vi "Drive Train.vi"() -> ()   [LabVIEW 2018]
uses:
  <vilib>/Rock Robotics/SystemInterfaces/DIO/FPGA_DIOChannel.ctl
  <vilib>/Rock Robotics/SystemInterfaces/AI/FPGA_AIChannel.ctl
  <vilib>/Rock Robotics/WPI/ThirdParty/Sensors/navX/_TypeDefs/FRIC_navX_DeviceNumbersTypeDef.ctl
  <vilib>/Rock Robotics/WPI/DriverStation/WPI_DriverStationRobotMode2.ctl
  <vilib>/Rock Robotics/WPI/ThirdParty/Phoenix-LabVIEW/Motor Controller/Controls/CTRE_Phoenix_MotorControl_NeutralMode.ctl
  <vilib>/Rock Robotics/WPI/Counter/WPI_CounterDigitalInputToDigitalSource.vi
  Times/Times Global.vi
  Drive Train Global.vi
  Robot Global Data.vi
  <vilib>/ptbypt/NI_PtbyPt.lvlib
panel:
  out "Cont Yaw Zero":dbl
  out "Loop 2":u32=30
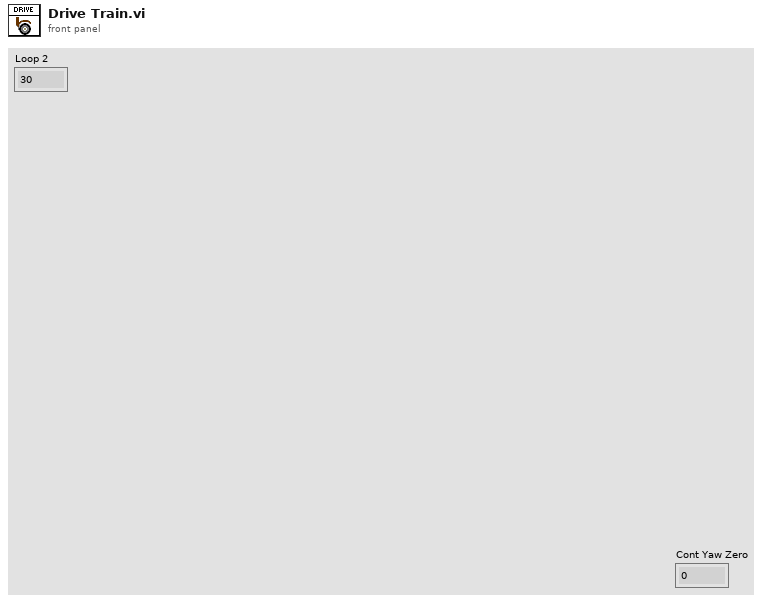
[diagram p1: front panel]
types:
  T1 = typedef "FPGA_AIChannel.ctl" = enum8{"AI 0", "AI 1", "AI 2", "AI 3", "AI MXP 0", "AI MXP 1", "AI MXP 2", "AI MXP 3", "Invalid"}
  T2 = typedef "FPGA_DIOChannel.ctl" = enum8{"DIO 0", "DIO 1", "DIO 2", "DIO 3", "DIO 4", "DIO 5", "DIO 6", "DIO 7", "DIO 8", "DIO 9", "DIO MXP 0", "DIO MXP 1", "DIO MXP 2", "DIO MXP 3", "DIO MXP 4", "DIO MXP 5", "DIO MXP 6", "DIO MXP 7", "DIO MXP 8", "DIO MXP 9", "DIO MXP 10", "DIO MXP 11", "DIO MXP 12", "DIO MXP 13", "DIO MXP 14", "DIO MXP 15", "SPI Port CS1", "SPI Port CS2", "SPI Port CS3", "SPI Port MISO", "SPI Port MOSI", "Invalid"}
  T3 = typedef "FRIC_navX_DeviceNumbersTypeDef.ctl" = enum16{"Dev0", "Dev1", "Dev2", "Dev3"}
  T4 = cluster{"Rollover":dbl, "Yaw":dbl, "Cont Yaw":dbl}
  T5 = typedef "CTRE_Phoenix_MotorControl_NeutralMode.ctl" = enum8{"EEPROMSetting", "Override to Coast", "Override to Brake"}
  T6 = typedef "WPI_MotorControlDeviceRef.ctl" = cluster{"DeviceStatus":errorcluster, "Type":T7, "PWM":cluster{"PWM Channel":T8, "DeadBand":T9}, "CAN":cluster{"Device Number":u8, "SetOutput VI Ref":variant, "GetOutput VI Ref":variant, "Enable VI Ref":variant, "Disable VI Ref":variant, "Data":variant}, "Invert":bool, "DIO PWM":cluster{"PWM \"Enable\" Channel":T8, "DIOChannel":T2, "PWM Rate":dbl}}
  T7 = typedef "WPI_MotorControlType.ctl" = enum16{"PWM", "CAN", "DIO PWM"}
  T8 = typedef "FPGA_DIOPWMChannel.ctl" = enum8{"PWM 0", "PWM 1", "PWM 2", "PWM 3", "PWM 4", "PWM 5", "PWM 6", "PWM 7", "PWM 8", "PWM 9", "PWM MXP 0", "PWM MXP 1", "PWM MXP 2", "PWM MXP 3", "PWM MXP 4", "PWM MXP 5", "PWM MXP 6", "PWM MXP 7", "PWM MXP 8", "PWM MXP 9", "Invalid"}
  T9 = typedef "WPI_PWMDeadband.ctl" = cluster{"Name":string, "maxPositivePwm":i32, "minPositivePwm":i32, "centerPwm":i32, "maxNegativePwm":i32, "minNegativePwm":i32, "angularRange":u16}
  T10 = typedef "WPI_DigitalInputDevRef.ctl" = cluster{"DevStatus":errorcluster, "DIO Channel":T2}
  T11 = typedef "WPI_PotentiometerDevRef.ctl" = cluster{"DevStatus":errorcluster, "Analog Channel":T1, "Invert Output":bool}
  T12 = typedef "FPGA_CounterEncoderSourceConvertionLVSourceType.ctl" = cluster{"DevStatus":errorcluster, "AnalogTriggerMode?":bool, "DigitalMode":cluster{"DIO Channel":T13}, "AnalogTriggerMode":cluster{"AnalogTriggerIndex":T14, "OutputType":T15}}
  T13 = typedef "FPGA_DIODigitalSourceChannel.ctl" = enum8{"DIO 0", "DIO 1", "DIO 2", "DIO 3", "DIO 4", "DIO 5", "DIO 6", "DIO 7", "DIO 8", "DIO 9", "DIO MXP 0", "DIO MXP 1", "DIO MXP 2", "DIO MXP 3", "DIO MXP 4", "DIO MXP 5", "DIO MXP 6", "DIO MXP 7", "DIO MXP 8", "DIO MXP 9", "DIO MXP 10", "DIO MXP 11", "DIO MXP 12", "DIO MXP 13", "DIO MXP 14", "DIO MXP 15", "SPI Port CS1", "SPI Port CS2", "SPI Port CS3", "SPI Port MISO", "SPI Port MOSI", "Disabled"}
  T14 = typedef "FPGA_AnalogTriggerIndex.ctl" = enum8{"Trig 0", "Trig 1", "Trig 2", "Trig 3", "Trig 4", "Trig 5", "Trig 6", "Trig 7", "Invalid"}
  T15 = typedef "FPGA_AnalogTriggerOutType.ctl" = enum16{"InWindow", "TriggerState", "Rising", "Falling"}
  T16 = typedef "WPI_EncoderDevRef.ctl" = cluster{"DevStatus":errorcluster, "EncoderIndex":T17, "CounterIndex":T18, "DistancePerCount":dbl, "Decoding Type":T19}
  T17 = typedef "FPGA_EncoderIdx.ctl" = enum8{"Enc 0", "Enc 1", "Enc 2", "Enc 3", "Enc 4", "Enc 5", "Enc 6", "Enc 7", "Invalid"}
  T18 = typedef "FPGA_CounterCtrSystemIndex.ctl" = enum8{"Ctr 0", "Ctr 1", "Ctr 2", "Ctr 3", "Ctr 4", "Ctr 5", "Ctr 6", "Ctr 7", "Invalid"}
  T19 = typedef "WPI_EncoderType.ctl" = enum16{"1x", "2x", "4x"}
  T20 = typedef "WPI_DriverStationRobotMode2.ctl" = enum16{"Autonomous Disabled", "Autonomous Enabled", "Teleop Disabled", "Teleop Enabled", "Disconnected", "Finish", "Test Disabled", "Test Enabled", "Emergency Stopped"}
  T21 = cluster{"FrontLeft":dbl, "FrontRight":dbl, "BackLeft":dbl, "BackRight":dbl}
  T22 = enum16{"Back Left", "Back Right", "Front Left", "Front Right"}
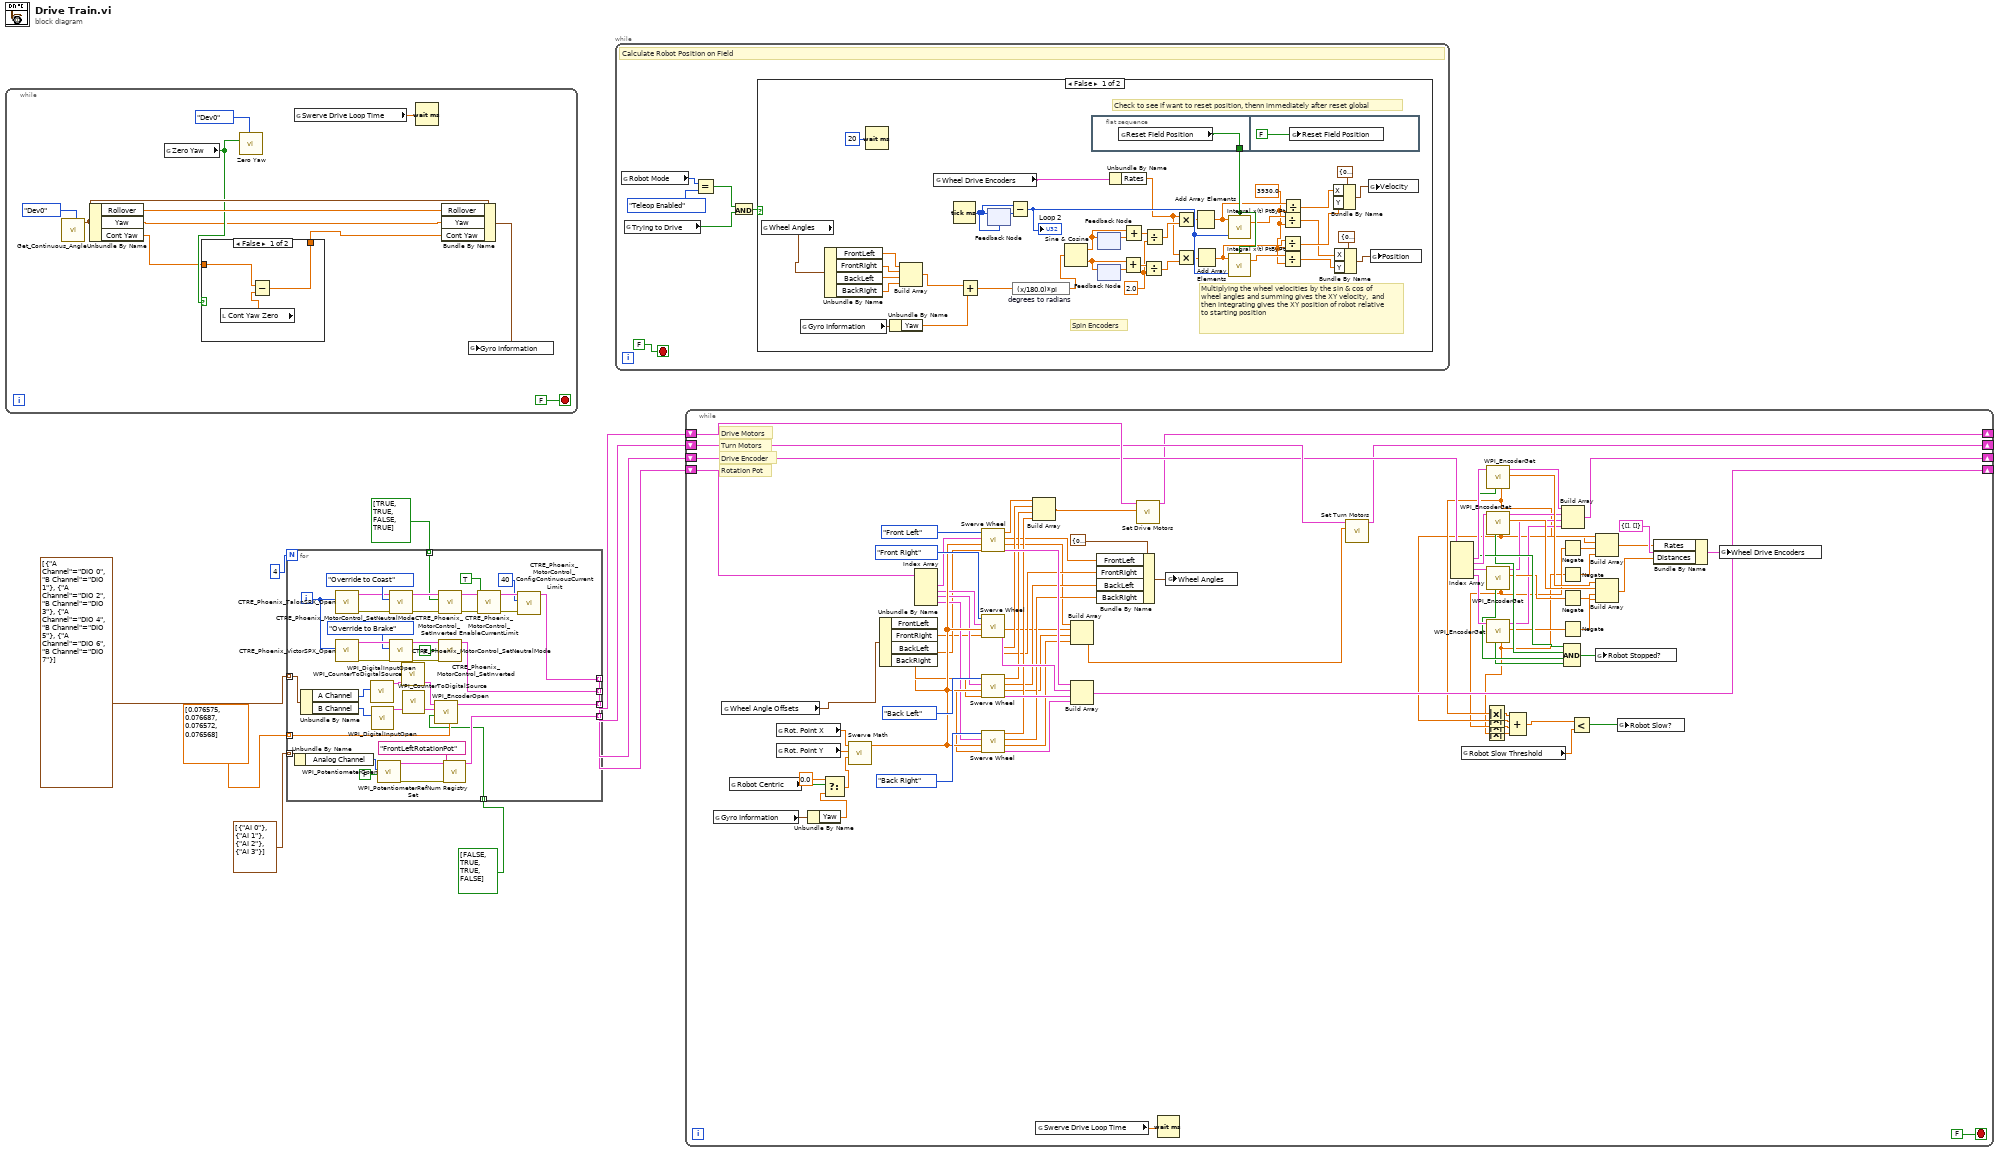
[diagram p0: block diagram]
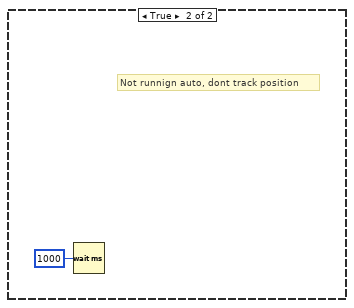
[diagram p2: hidden frame]
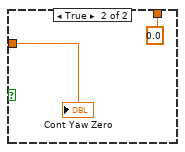
[diagram p3: hidden frame]
diagram:
  n1 = while {
    stop <- FALSE stop-if-true
    n2 = call <vilib>:"Get_Continuous_Angle.vi"("Device Number"=FRIC_navX_DeviceNumbersTypeDef."Dev0") -> ("Continuous Angle"=w15:T4)  [unwired: 10 in]
    n3 = Unbundle By Name(w15) -> ("Rollover"=w16:dbl, "Yaw"=w12:dbl, "Cont Yaw"=w13:dbl)
    n4 = global read "Drive Train Global.vi" "Zero Yaw"() -> (w14:bool)
    n5 = case shown="False" w14 {
      tunnel: w13 -> [w24 w26]
      tunnel: [w23 0.0] -> w11
      frame False {
        n6 = local read "Cont Yaw Zero"() -> (w22:dbl)
        n7 = Subtract(x=w24, y=w22) -> (x-y=w23:dbl)
      }
      frame True {
        "Cont Yaw Zero" <- w26
      }
    }
    n8 = call <vilib>:"Zero Yaw.vi"("Device Number"=FRIC_navX_DeviceNumbersTypeDef."Dev0", "Zero"=w14) -> ()  [unwired: 10 in]
    n9 = global read "Times Global.vi" "Swerve Drive Loop Time"() -> (w19:dbl)
    n10 = Wait (ms)(milliseconds to wait=w19) -> ()  [unwired: 1 out]
    n11 = Bundle By Name(cluster=w15, "Rollover"=w16, "Yaw"=w12, "Cont Yaw"=w11) -> (w17:T4)
    n12 = global write "Drive Train Global.vi" "Gyro Information"(w17) -> ()
  }
  n13 = for {
    N: 4 -> [_]
    tunnel: cluster{"A Channel":T2, "B Channel":T2}[] [{"A Channel"=enum."DIO 0", "B Channel"=enum."DIO 1"}, {"A Channel"=enum."DIO 2", "B Channel"=enum."DIO 3"}, {"A Channel"=enum."DIO 4", "B Channel"=enum."DIO 5"}, {"A Channel"=enum."DIO 6", "B Channel"=enum."DIO 7"}] -> [w44] mode=indexing
    tunnel: cluster{"Analog Channel":T1}[] [{"Analog Channel"=enum."AI 0"}, {"Analog Channel"=enum."AI 1"}, {"Analog Channel"=enum."AI 2"}, {"Analog Channel"=enum."AI 3"}] -> [w41] mode=indexing
    tunnel: dbl[] [0.076575, 0.076687, 0.076572, 0.076568] -> [w39] mode=indexing
    tunnel: [w28] -> w6 mode=indexing
    tunnel: [w38] -> w5 mode=indexing
    tunnel: [w37] -> w4 mode=indexing
    tunnel: [w36] -> w3 mode=indexing
    tunnel: bool[] [TRUE, TRUE, FALSE, TRUE] -> [w35] mode=indexing
    tunnel: bool[] [FALSE, TRUE, TRUE, FALSE] -> [w27] mode=indexing
    i -> [w45]
    n14 = Unbundle By Name(w41) -> ("Analog Channel"=w40:T1)
    n15 = Unbundle By Name(w44) -> ("A Channel"=w43:T2, "B Channel"=w42:T2)
    n16 = call <vilib>:"CTRE_Phoenix_TalonSRX_Open.vi"("Device Number"=w45) -> ("error out"=w46:errorcluster, "CAN Talon SRX Ref"=w47:T6)  [unwired: 9 in]
    n17 = call <vilib>:"CTRE_Phoenix_VictorSPX_Open.vi"("Device Number"=w45) -> ("error out"=w56:errorcluster, "CAN Talon SRX Ref"=w55:T6)  [unwired: 9 in]
    n18 = call <vilib>:"WPI_DigitalInputOpen.vi"("DIO Channel"=w43) -> ("DigitalInputDevRef"=w63:T10)  [unwired: 1 in, 9 out]
    n19 = call <vilib>:"WPI_DigitalInputOpen.vi"("DIO Channel"=w42) -> ("DigitalInputDevRef"=w62:T10)  [unwired: 1 in, 9 out]
    n20 = call <vilib>:"WPI_PotentiometerOpen.vi"("Invert Output"=FALSE, "Analog Channel"=w40) -> ("error out"=w58:errorcluster, "PotDevRef"=w59:T11)  [unwired: 8 in]
    n21 = call <vilib>:"CTRE_Phoenix_MotorControl_SetNeutralMode.vi"("error in (no error)"=w46, "Motor Control Neutral Mode"=CTRE_Phoenix_MotorControl_NeutralMode."Override to Coast", "PhoenixMotorControlDevRef"=w47) -> ("error out"=w49:errorcluster, "PhoenixMotorControlDevRef"=w50:T6)  [unwired: 7 in]
    n22 = call <vilib>:"CTRE_Phoenix_MotorControl_SetNeutralMode.vi"("error in (no error)"=w56, "Motor Control Neutral Mode"=CTRE_Phoenix_MotorControl_NeutralMode."Override to Brake", "PhoenixMotorControlDevRef"=w55) -> ("error out"=w53:errorcluster, "PhoenixMotorControlDevRef"=w52:T6)  [unwired: 7 in]
    n23 = call-poly <vilib>:"WPI_CounterToDigitalSource.vi"("DigitalInputDevRef"=w63) -> ("Digital Source"=w64:T12)  [unwired: 6 out]
    n24 = call-poly <vilib>:"WPI_CounterToDigitalSource.vi"("DigitalInputDevRef"=w62) -> ("Digital Source"=w61:T12)  [unwired: 6 out]
    n25 = call <vilib>:"WPI_EncoderOpen.vi"("DistancePerCount"=w39, "Invert Direction (False)"=w27, "BSource"=w61, "ASource"=w64) -> ("EncoderDevRef"=w37:T16)  [unwired: 4 in, 3 out]
    n26 = call <vilib>:"CTRE_Phoenix_MotorControl_SetInverted.vi"("error in (no error)"=w49, "Invert?"=w35, "PhoenixMotorControlDevRef"=w50) -> ("error out"=w34:errorcluster, "PhoenixMotorControlDevRef"=w33:T6)  [unwired: 7 in]
    n27 = call <vilib>:"CTRE_Phoenix_MotorControl_SetInverted.vi"("error in (no error)"=w53, "Invert?"=FALSE, "PhoenixMotorControlDevRef"=w52) -> ("PhoenixMotorControlDevRef"=w38:T6)  [unwired: 7 in, 1 out]
    n28 = call <vilib>:"WPI_PotentiometerRefNum Registry Set.vi"("error in (no error)"=w58, "refnum name"="FrontLeftRotationPot", "PotDevRef"=w59) -> ("PotDevRef"=w36:T11)  [unwired: 7 in, 1 out]
    n29 = call <vilib>:"CTRE_Phoenix_MotorControl_EnableCurrentLimit.vi"("error in (no error)"=w34, "Enable Current Limit?"=TRUE, "PhoenixMotorControlDevRef"=w33) -> ("error out"=w31:errorcluster, "PhoenixMotorControlDevRef"=w30:T6)  [unwired: 7 in]
    n30 = call <vilib>:"CTRE_Phoenix_MotorControl_ConfigContinuousCurrentLimit.vi"("error in (no error)"=w31, "Continuous Current Limit (Amps)"=40, "PhoenixMotorControlDevRef"=w30) -> ("PhoenixMotorControlDevRef"=w28:T6)  [unwired: 7 in, 1 out]
  }
  n31 = while {
    stop <- FALSE stop-if-true
    # "Calculate Robot Position on Field"
    n32 = global read "Robot Global Data.vi" "Robot Mode"() -> (w69:T20)
    n33 = global read "Robot Global Data.vi" "Trying to Drive"() -> (w66:bool)
    n34 = Equal?(x=w69, y=WPI_DriverStationRobotMode2."Teleop Enabled") -> (x = y?=w65:bool)
    n35 = And(x=w65, y=w66) -> (x .and. y?=w67:bool)
    n36 = case shown="False" w67 {
      frame False {
        w90 = 3930.0 ("y")
        w100 = 2.0
        # "Check to see if want to reset position, thenn immediately after reset global"
        # "Spin Encoders"
        # "Multiplying the wheel velocities by the sin & cos of wheel angles and summing gives the XY velocity,  and then integrating gives the XY position of robot relative to starting position"
        n37 = global read "Drive Train Global.vi" "Wheel Angles"() -> (w88:T21)
        n38 = global read "Drive Train Global.vi" "Gyro Information"() -> (w81:T4)
        n39 = Unbundle By Name(w88) -> ("FrontLeft"=w87:dbl, "FrontRight"=w86:dbl, "BackLeft"=w85:dbl, "BackRight"=w84:dbl)
        n40 = Wait (ms)(milliseconds to wait=u32 20) -> ()  [unwired: 1 out]
        n41 = Unbundle By Name(w81) -> ("Yaw"=w80:dbl)
        n42 = Build Array(w87, w86, w85, w84) -> (w83:dbl[])
        n43 = global read "Drive Train Global.vi" "Wheel Drive Encoders"() -> (w82:cluster{"Rates":dbl[], "Distances":dbl[]})
        n44 = Tick Count (ms)() -> (millisecond timer value=w96:u32)
        n45 = Add(x=w83, y=w80) -> (x+y=w89:dbl[])
        n46 = feedback #1(w96) -> (w111:u32)
        n47 = feedback-in #1(w96) -> ()
        n48 = Subtract(x=w96, y=w111) -> (x-y=w110:u32)
        "Loop 2" <- w110
        n49 = expression code="(x/180.0)*pi" "degrees to radians"(w89) -> (w95:dbl[])
        n50 = Sine & Cosine(0:w95) -> (1:w106:dbl[], 2:w101:dbl[])
        n51 = flat-sequence {
          tunnel: [w112] -> w98
          frame #0 {
            n52 = global read "Drive Train Global.vi" "Reset Field Position"() -> (w112:bool)
          }
          frame #1 {
            n53 = global write "Drive Train Global.vi" "Reset Field Position"(FALSE) -> ()
          }
        }
        n54 = feedback #2() -> (w107:dbl[])  [unwired: 1 in]
        n55 = feedback-in #2(w106) -> ()
        n56 = feedback #3() -> (w102:dbl[])  [unwired: 1 in]
        n57 = feedback-in #3(w101) -> ()
        n58 = Unbundle By Name(w82) -> ("Rates"=w97:dbl[])
        n59 = Add(x=w101, y=w102) -> (x+y=w103:dbl[])
        n60 = Add(x=w106, y=w107) -> (x+y=w104:dbl[])
        n61 = Divide(x=w103, y=w100) -> (x/y=w99:dbl[])
        n62 = Divide(x=w104, y=w100) -> (x/y=w105:dbl[])
        n63 = Multiply(x=w97, y=w105) -> (x*y=w109:dbl[])
        n64 = Multiply(x=w97, y=w99) -> (x*y=w108:dbl[])
        n65 = Add Array Elements(numeric array=w109) -> (sum=w93:dbl)
        n66 = Add Array Elements(numeric array=w108) -> (sum=w92:dbl)
        n67 = call <vilib>:"Integral x(t) PtByPt.vi"("initialize"=w98, "dt"=w110, "x"=w93) -> ("integral x(t)"=w94:dbl)  [unwired: 1 in, 1 out]
        n68 = call <vilib>:"Integral x(t) PtByPt.vi"("initialize"=w98, "dt"=w110, "x"=w92) -> ("integral x(t)"=w91:dbl)  [unwired: 1 in, 1 out]
        n69 = Divide(x=w94, y=w90) -> (x/y=w74:dbl)
        n70 = Divide(x=w92, y=w90) -> (x/y=w77:dbl)
        n71 = Divide(x=w91, y=w90) -> (x/y=w73:dbl)
        n72 = Divide(x=w93, y=w90) -> (x/y=w79:dbl)
        n73 = Bundle By Name(cluster=cluster{"X":dbl, "Y":dbl} {"X"=0.0, "Y"=0.0} ("Position"), "X"=w79, "Y"=w77) -> (w71:cluster{"X":dbl, "Y":dbl})
        n74 = Bundle By Name(cluster=cluster{"X":dbl, "Y":dbl} {"X"=0.0, "Y"=0.0} ("Position"), "X"=w74, "Y"=w73) -> (w75:cluster{"X":dbl, "Y":dbl})
        n75 = global write "Drive Train Global.vi" "Velocity"(w71) -> ()
        n76 = global write "Drive Train Global.vi" "Position"(w75) -> ()
      }
      frame True {
        # "Not runnign auto, dont track position"
        n77 = Wait (ms)(milliseconds to wait=u32 1000) -> ()  [unwired: 1 out]
      }
    }
  }
  n78 = while {
    shift-right: [w195] -> _
    shift-left: w6 -> [w199]
    shift-right: [w194] -> _
    shift-left: w5 -> [w198]
    shift-right: [w193] -> _
    shift-left: w4 -> [w197]
    shift-right: [w192] -> _
    shift-left: w3 -> [w196]
    stop <- FALSE stop-if-true
    # "Rotation Pot"
    # "Drive Encoder"
    # "Turn Motors"
    # "Drive Motors"
    n79 = global read "Drive Train Global.vi" "Gyro Information"() -> (w186:T4)
    n80 = global read "Drive Train Global.vi" "Wheel Angle Offsets"() -> (w153:T21)
    n81 = global read "Drive Train Global.vi" "Robot Centric"() -> (w156:bool)
    n82 = global read "Drive Train Global.vi" "Rot. Point X"() -> (w185:dbl)
    n83 = global read "Drive Train Global.vi" "Rot. Point Y"() -> (w184:dbl)
    n84 = Unbundle By Name(w186) -> ("Yaw"=w154:dbl)
    n85 = Select(t=0.0, s=w156, f=w154) -> (s? t:f=w157:dbl)
    n86 = call "Swerve Math.vi"("Yaw"=w157, "Rot. Point Y"=w184, "Rot. Point X"=w185) -> ("Swerve Math Ouput"=w187:dbl[])  [unwired: 8 in]
    n87 = Unbundle By Name(w153) -> ("FrontLeft"=w161:dbl, "FrontRight"=w160:dbl, "BackLeft"=w159:dbl, "BackRight"=w158:dbl)
    n88 = Index Array(array=w196) -> (element #1=w183:T11, element #2=w182:T11, element #3=w181:T11, element #4=w180:T11)  [unwired: 4 in]
    n89 = call "Swerve Wheel.vi"("Wheel Angle Offset"=w161, "Inputs"=w187, "Pot Ref In"=w183, "Wheel"=T22."Front Left") -> ("Pot Ref Out"=w176:T11, "Motor Output"=w165:dbl, "Wheel Angle"=w170:dbl, "Speed"=w175:dbl)  [unwired: 4 in]
    n90 = call "Swerve Wheel.vi"("Wheel Angle Offset"=w160, "Inputs"=w187, "Pot Ref In"=w182, "Wheel"=T22."Front Right") -> ("Pot Ref Out"=w177:T11, "Motor Output"=w164:dbl, "Wheel Angle"=w169:dbl, "Speed"=w174:dbl)  [unwired: 4 in]
    n91 = call "Swerve Wheel.vi"("Wheel Angle Offset"=w159, "Inputs"=w187, "Pot Ref In"=w181, "Wheel"=T22."Back Left") -> ("Pot Ref Out"=w178:T11, "Motor Output"=w163:dbl, "Wheel Angle"=w168:dbl, "Speed"=w173:dbl)  [unwired: 4 in]
    n92 = call "Swerve Wheel.vi"("Wheel Angle Offset"=w158, "Inputs"=w187, "Pot Ref In"=w180, "Wheel"=T22."Back Right") -> ("Pot Ref Out"=w179:T11, "Motor Output"=w162:dbl, "Wheel Angle"=w167:dbl, "Speed"=w172:dbl)  [unwired: 4 in]
    n93 = Build Array(w175, w174, w173, w172) -> (w151:dbl[])
    n94 = global read "Times Global.vi" "Swerve Drive Loop Time"() -> (w200:dbl)
    n95 = Build Array(w165, w164, w163, w162) -> (w152:dbl[])
    n96 = Build Array(w176, w177, w178, w179) -> (w192:T11[])
    n97 = Bundle By Name(cluster=T21 {"FrontLeft"=0.0, "FrontRight"=0.0, "BackLeft"=0.0, "BackRight"=0.0} ("Wheel Angles"), "FrontLeft"=w170, "FrontRight"=w169, "BackLeft"=w168, "BackRight"=w167) -> (w166:T21)
    n98 = call "Set Drive Motors.vi"("appended array"=w151, "Motors In"=w199) -> ("Motors Out"=w195:T6[])  [unwired: 9 in]
    n99 = Wait (ms)(milliseconds to wait=w200) -> ()  [unwired: 1 out]
    n100 = global write "Drive Train Global.vi" "Wheel Angles"(w166) -> ()
    n101 = call "Set Turn Motors.vi"("appended array"=w152, "Motors In"=w198) -> ("Motors Out"=w194:T6[])  [unwired: 9 in]
    n102 = Index Array(array=w197) -> (element #1=w150:T16, element #2=w149:T16, element #3=w148:T16, element #4=w147:T16)  [unwired: 4 in]
    n103 = global read "Drive Train Global.vi" "Robot Slow Threshold"() -> (w115:dbl)
    n104 = call <vilib>:"WPI_EncoderGet.vi"("EncoderDevRef"=w150) -> ("Distance"=w130:dbl, "EncoderDevRef"=w129:T16, "Rate"=w120:dbl, "Stopped"=w141:bool)  [unwired: 5 in, 2 out]
    n105 = Absolute Value(x=w120) -> (abs(x)=w124:dbl)
    n106 = call <vilib>:"WPI_EncoderGet.vi"("EncoderDevRef"=w149) -> ("Distance"=w134:dbl, "EncoderDevRef"=w128:T16, "Rate"=w119:dbl, "Stopped"=w140:bool)  [unwired: 5 in, 2 out]
    n107 = Absolute Value(x=w119) -> (abs(x)=w123:dbl)
    n108 = call <vilib>:"WPI_EncoderGet.vi"("EncoderDevRef"=w148) -> ("Distance"=w133:dbl, "EncoderDevRef"=w127:T16, "Rate"=w118:dbl, "Stopped"=w139:bool)  [unwired: 5 in, 2 out]
    n109 = Absolute Value(x=w118) -> (abs(x)=w122:dbl)
    n110 = call <vilib>:"WPI_EncoderGet.vi"("EncoderDevRef"=w147) -> ("Distance"=w136:dbl, "EncoderDevRef"=w126:T16, "Rate"=w117:dbl, "Stopped"=w138:bool)  [unwired: 5 in, 2 out]
    n111 = Absolute Value(x=w117) -> (abs(x)=w121:dbl)
    n112 = Compound Arithmetic op=ADD(w124, w123, w122, w121) -> (w125:dbl)
    n113 = Negate(x=w118) -> (-x=w131:dbl)
    n114 = Negate(x=w117) -> (-x=w137:dbl)
    n115 = Negate(x=w133) -> (-x=w132:dbl)
    n116 = Negate(x=w136) -> (-x=w135:dbl)
    n117 = Build Array(w129, w128, w127, w126) -> (w193:T16[])
    n118 = Compound Arithmetic op=AND(w141, w140, w139, w138) -> (w142:bool)
    n119 = Less?(x=w125, y=w115) -> (x < y?=w116:bool)
    n120 = Build Array(w120, w119, w131, w137) -> (w144:dbl[])
    n121 = Build Array(w130, w134, w132, w135) -> (w143:dbl[])
    n122 = global write "Drive Train Global.vi" "Robot Stopped?"(w142) -> ()
    n123 = global write "Drive Train Global.vi" "Robot Slow?"(w116) -> ()
    n124 = Bundle By Name(cluster=cluster{"Rates":dbl[], "Distances":dbl[]} {"Rates"=[], "Distances"=[]} ("Wheel Drive Encoders"), "Rates"=w144, "Distances"=w143) -> (w146:cluster{"Rates":dbl[], "Distances":dbl[]})
    n125 = global write "Drive Train Global.vi" "Wheel Drive Encoders"(w146) -> ()
  }
